vi "UninitDL.vi"(2 "Container State":T1, 3 "Display State":T2={"param"=[], "positions"=[0.0, 0.0, 0.0], "CellsI"=enum."5", "CellsIII"=enum."7", "DLI short "=refnum, "DLIII short"=refnum, "DLII long"=refnum, "step,ps"=100, " preset pos"=[]}) -> ()   [LabVIEW 2019, in "ControlDL.xctl"]
uses:
  ControlDL.xctl
  stateDL.ctl
  controls/CellsSDI.ctl
  controls/CellBoolean.ctl
  controls/CellsSDIII.ctl
  <vilib>/_xctls/Container State.ctl
  <vilib>/_xctls/XControlSupport.lvlib
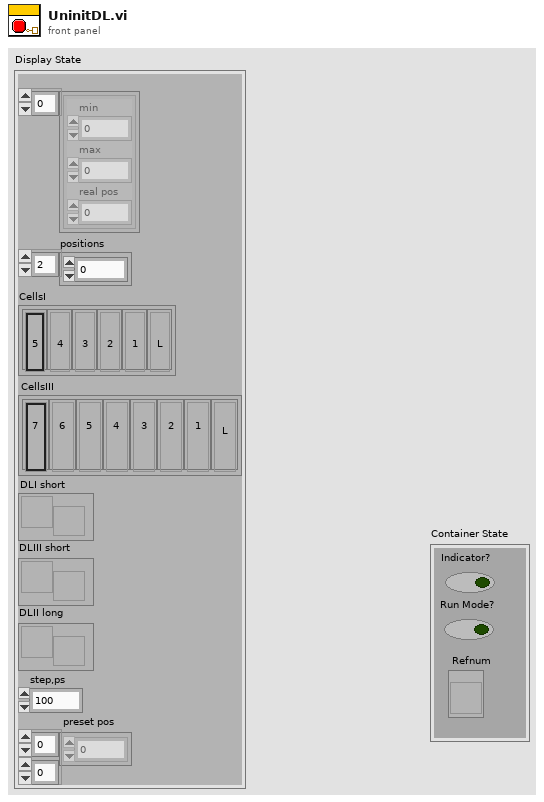
[diagram p1: front panel]
types:
  T1 = typedef "XControlSupport.lvlib/Container State.ctl" = cluster{"Indicator?":bool, "Run Mode?":bool, " Refnum":refnum<vi>}
  T2 = typedef "ControlDL.xctl/stateDL.ctl" = cluster{"param":cluster{"min":dbl, "max":dbl, "real pos":dbl}[], "positions":dbl[], "CellsI":T3, "CellsIII":T4, "DLI short ":refnum<user-event>, "DLIII short":refnum<user-event>, "DLII long":refnum<user-event>, "step,ps":i32, " preset pos":dbl[][]}
  T3 = typedef "CellsSDI.ctl" = enum32{"5", "4", "3", "2", "1", "L"}
  T4 = typedef "CellsSDIII.ctl" = enum32{"7", "6", "5", "4", "3", "2", "1", "L"}
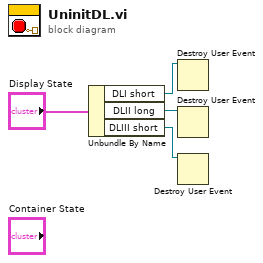
[diagram p0: block diagram]
diagram:
  n1 = Unbundle By Name("Display State") -> ("DLI short"=w3:refnum<user-event>, "DLII long"=w2:refnum<user-event>, "DLIII short"=w1:refnum<user-event>)
  n2 = Destroy User Event(user event=w3) -> ()  [unwired: 1 in, 1 out]
  n3 = Destroy User Event(user event=w2) -> ()  [unwired: 1 in, 1 out]
  n4 = Destroy User Event(user event=w1) -> ()  [unwired: 1 in, 1 out]
